vi "newEnergyAxis.vi"(8 "error in (no error)":errorcluster, 11 "Cam Cluster out in":T1={"incident ANGLE COMPENSATION"=[], "dp/B [MeV/C/B]"=[], "charge compensation"=[], "Momentum [MeV/C]"=[], "energyDependence Input"=[], "pixel angle (y)"=[], "dp [MeV/C/] "=[], "angle 2Dfor spectrumj"=[], "dp [MeV/C] 2D"=[], "charge compensation 2D"=[], "Screen&Camera 2"={"Screen Orientation"="Regular", "Screen angle"="Flat", "Lens"=enum."FL3M14-f8x08(2x2)", "Calibration (mm/pix)"=0.231}, "ROI info"={"npix-X"=692, "npix-Y"=516, "Left [pix]"=88.0, "Top [pix]"=368.0}, "Y 2D full angle"=array96x262[25152 elements], "calib pixel"={"y1(pixel)"=array[262 elements], "y2(pixel)"=array[262 elements], "dp/B [MeV/C/B] (pixel)"=array[262 elements], "energyDependence Input(pixel)"=array[262 elements], "bending angle [deg](pixel)"=array[262 elements], "total path(pixel)"=array[262 elements], "pixel angle (y)(pixel)"=array[262 elements], "energy dependence (pixel)"=array[262 elements], "charge compensation (pixel)"=array[262 elements], "Momentum [MeV/C](pixel)"=array[262 elements], "angular compensation(pixel)"=array[262 elements]}, "2D"={"dp"=array96x262[25152 elements], "chargeCompensation"=array96x262[25152 elements], "angle"=array96x262[25152 elements], "Momentum"=[]}, "UserROI"={"Width"=262.0, "Hight"=96.0, "OffsetX"=88.0, "OffsetY"=188.0}, "final"={"X"=[], "xi"=[], "delta momentum"=0.0, "Y"=array96x262[25152 elements], "yi"=[], "angle (Y)"=[-5.5913315463290765, -5.505311061000937, -5.419290575672798, -5.333270090344658, -5.247249605016518, -5.161229119688378, -5.075208634360239, -4.989188149032099, -4.903167663703959, -4.817147178375819, -4.73112669304768, -4.64510620771954, -4.5590857223914005, -4.4730652370632615, -4.387044751735122, -4.301024266406982, -4.215003781078842, -4.128983295750703, -4.042962810422563, -3.956942325094423, -3.8709218397662837, -3.784901354438144, -3.6988808691100044, -3.612860383781865, -3.526839898453725, -3.4408194131255856, -3.3547989277974457, -3.2687784424693063, -3.1827579571411664, -3.096737471813027, -3.010716986484887, -2.9246965011567476, -2.838676015828608, -2.7526555305004683, -2.666635045172329, -2.580614559844189, -2.4945940745160495, -2.4085735891879096, -2.32255310385977, -2.2365326185316303, -2.150512133203491, -2.064491647875351, -1.9784711625472116, -1.892450677219072, -1.8064301918909322, -1.7204097065627926, -1.634389221234653, -1.5483687359065132, -1.4623482505783738, -1.3763277652502341, -1.2903072799220945, -1.2042867945939548, -1.1182663092658152, -1.0322458239376755, -0.9462253386095358, -0.8602048532813962, -0.7741843679532566, -0.688163882625117, -0.6021433972969773, -0.5161229119688376, -0.43010242664069803, -0.34408194131255837, -0.2580614559844187, -0.1720409706562791, -0.08602048532813945, 1.8735013540549517e-16, 0.08602048532813983, 0.17204097065627946, 0.2580614559844191, 0.34408194131255876, 0.43010242664069837, 0.5161229119688381, 0.6021433972969776, 0.6881638826251173, 0.774184367953257, 0.8602048532813966, 0.9462253386095363, 1.032245823937676, 1.1182663092658156, 1.2042867945939553, 1.2903072799220947, 1.3763277652502344, 1.462348250578374, 1.5483687359065137, 1.6343892212346534, 1.720409706562793, 1.8064301918909327, 1.8924506772190723, 1.978471162547212, 2.0644916478753514, 2.1505121332034913, 2.2365326185316308, 2.3225531038597707, 2.40857358918791, 2.49459407451605, 2.5806145598441894], "delta angle"=0.08602048532813988, "scale delta angle"=1.0476789973922933, "intraX"=0.0, "intraY"=96.0, "mask"=[]}, "B[T]"=0.07999999999999999, "index"=0.0}) -> (0 "error out":errorcluster, 3 "output cluster":T1={"incident ANGLE COMPENSATION"=[], "dp/B [MeV/C/B]"=[], "charge compensation"=[], "Momentum [MeV/C]"=[], "energyDependence Input"=[], "pixel angle (y)"=[], "dp [MeV/C/] "=[], "angle 2Dfor spectrumj"=[], "dp [MeV/C] 2D"=[], "charge compensation 2D"=[], "Screen&Camera 2"={"Screen Orientation"="Regular", "Screen angle"="Flat", "Lens"=enum."FL1-f8x08", "Calibration (mm/pix)"=1.0}, "ROI info"={"npix-X"=0, "npix-Y"=0, "Left [pix]"=0.0, "Top [pix]"=0.0}, "Y 2D full angle"=[], "calib pixel"={"y1(pixel)"=[], "y2(pixel)"=[], "dp/B [MeV/C/B] (pixel)"=[], "energyDependence Input(pixel)"=[], "bending angle [deg](pixel)"=[], "total path(pixel)"=[], "pixel angle (y)(pixel)"=[], "energy dependence (pixel)"=[], "charge compensation (pixel)"=[], "Momentum [MeV/C](pixel)"=[], "angular compensation(pixel)"=[]}, "2D"={"dp"=[], "chargeCompensation"=[], "angle"=[], "Momentum"=[]}, "UserROI"={"Width"=0.0, "Hight"=0.0, "OffsetX"=0.0, "OffsetY"=0.0}, "final"={"X"=[], "xi"=[], "delta momentum"=0.0, "Y"=[], "yi"=[], "angle (Y)"=[], "delta angle"=0.0, "scale delta angle"=0.0, "intraX"=0.0, "intraY"=0.0, "mask"=[]}, "B[T]"=0.0, "index"=0.0})   [LabVIEW 2020]
uses:
  calib_Sub_Typdef.ctl
  ScreenCam2_TypDEf.ctl
  CamAndObj_TypDEf.ctl
  ROIInfo_TypDef.ctl
  calibPixel.ctl
  2DTypDef.ctl
  CamRoiTypDef.ctl
  finalCalibTypdef.ctl
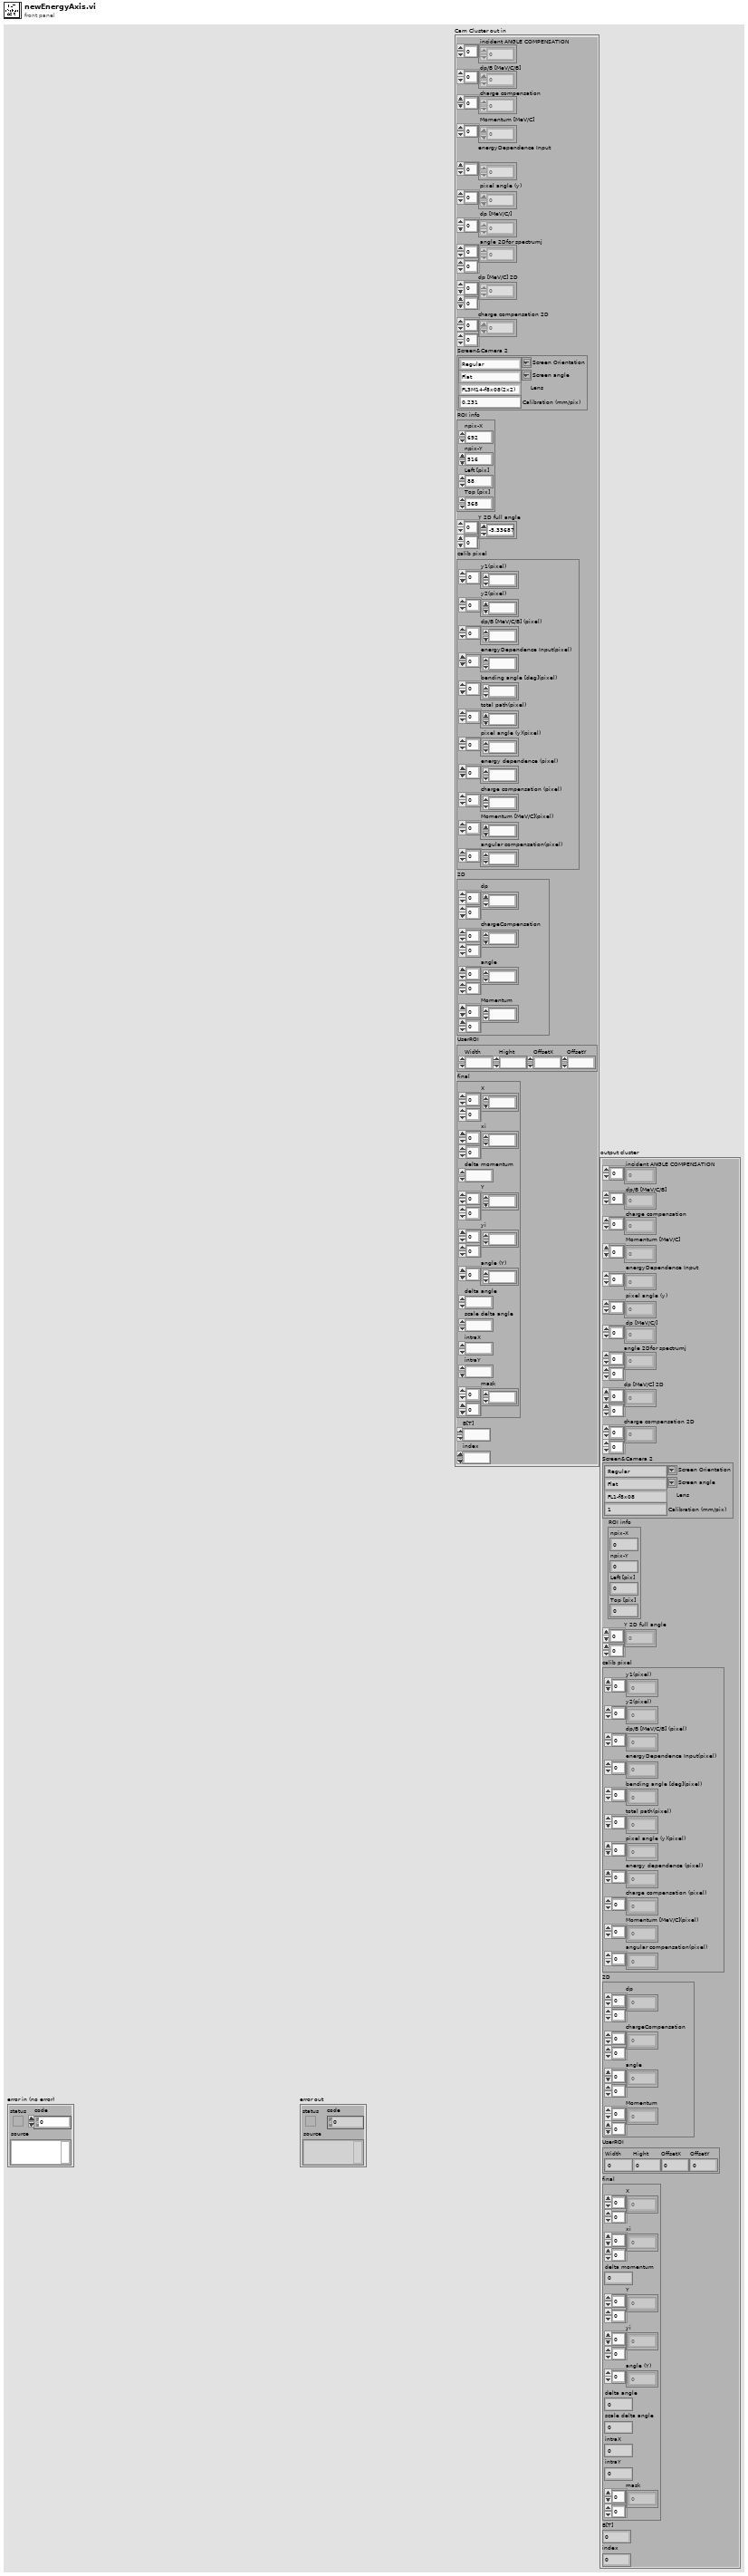
[diagram p1: front panel]
types:
  T1 = typedef "calib_Sub_Typdef.ctl" = cluster{"incident ANGLE COMPENSATION":dbl[], "dp/B [MeV/C/B]":dbl[], "charge compensation":dbl[], "Momentum [MeV/C]":dbl[], "energyDependence Input":dbl[], "pixel angle (y)":dbl[], "dp [MeV/C/] ":dbl[], "angle 2Dfor spectrumj":dbl[][], "dp [MeV/C] 2D":dbl[][], "charge compensation 2D":dbl[][], "Screen&Camera 2":T2, "ROI info":T4, "Y 2D full angle":dbl[][], "calib pixel":T5, "2D":T6, "UserROI":T7, "final":T8, "B[T]":dbl, "index":dbl}
  T2 = typedef "ScreenCam2_TypDEf.ctl" = cluster{"Screen Orientation":string, "Screen angle":string, "Lens":T3, "Calibration (mm/pix)":dbl}
  T3 = typedef "CamAndObj_TypDEf.ctl" = enum16{"FL1-f8x08", "FL1-f8x06", "FL1-f8", "ch300-f50", "FL2G-f8", "FL3M14-f8", "FL3M14-f8x08", "FL3M14-f8x08(2x2)"}
  T4 = typedef "ROIInfo_TypDef.ctl" = cluster{"npix-X":i32, "npix-Y":i32, "Left [pix]":dbl, "Top [pix]":dbl}
  T5 = typedef "calibPixel.ctl" = cluster{"y1(pixel)":dbl[], "y2(pixel)":dbl[], "dp/B [MeV/C/B] (pixel)":dbl[], "energyDependence Input(pixel)":dbl[], "bending angle [deg](pixel)":dbl[], "total path(pixel)":dbl[], "pixel angle (y)(pixel)":dbl[], "energy dependence (pixel)":dbl[], "charge compensation (pixel)":dbl[], "Momentum [MeV/C](pixel)":dbl[], "angular compensation(pixel)":dbl[]}
  T6 = typedef "2DTypDef.ctl" = cluster{"dp":dbl[][], "chargeCompensation":dbl[][], "angle":dbl[][], "Momentum":dbl[][]}
  T7 = typedef "CamRoiTypDef.ctl" = cluster{"Width":dbl, "Hight":dbl, "OffsetX":dbl, "OffsetY":dbl}
  T8 = typedef "finalCalibTypdef.ctl" = cluster{"X":dbl[][], "xi":dbl[][], "delta momentum":dbl, "Y":dbl[][], "yi":dbl[][], "angle (Y)":dbl[], "delta angle":dbl, "scale delta angle":dbl, "intraX":dbl, "intraY":dbl, "mask":dbl[][]}
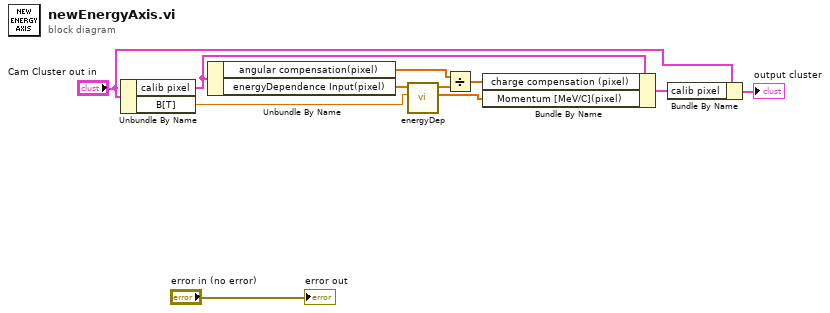
[diagram p0: block diagram]
diagram:
  n1 = Unbundle By Name("Cam Cluster out in") -> ("calib pixel"=w6:T5, "B[T]"=w2:dbl)
  n2 = Unbundle By Name(w6) -> ("angular compensation(pixel)"=w8:dbl[], "energyDependence Input(pixel)"=w11:dbl[])
  n3 = call "energyDep.vi"("B [T]"=w2, "energy Dep in"=w11) -> ("Momentum [MeV/C]"=w10:dbl[], "energy dependence"=w7:dbl[])  [unwired: 8 in]
  n4 = Divide(x=w8, y=w7) -> (x/y=w9:dbl[])
  n5 = Bundle By Name(cluster=w6, "charge compensation (pixel)"=w9, "Momentum [MeV/C](pixel)"=w10) -> (w4:T5)
  n6 = Bundle By Name(cluster="Cam Cluster out in", "calib pixel"=w4) -> (→"output cluster":T1)
  "error out" <- "error in (no error)"
